vi "pmu_Write ROCOF Detector Settings.vi"(8 "error in (no error)":errorcluster, 10 "ROCOF detector settings":T1={"ROCOF window width"=2}, 11 "system info in":refnum<class "PMU System Info.lvclass">) -> (0 "error out":errorcluster, 3 "system info out":refnum<class "PMU System Info.lvclass">)   [LabVIEW 2013, in "NI_EP_PMU.lvlib" / "PMU System Info.lvclass"]
uses:
  <vilib>/addons/Electrical Power/PMU/Common/Classes/PMU System Info/PMU System Info.lvclass
  <vilib>/addons/Electrical Power/PMU/Common/Controls/pmu_ROCOF Detector Settings.ctl
  <vilib>/addons/Electrical Power/PMU/Common/Classes/PMU System Info/PMU System Info.lvclass/PMU System Info.ctl
  <vilib>/addons/Electrical Power/PMU/NI_EP_PMU.lvlib
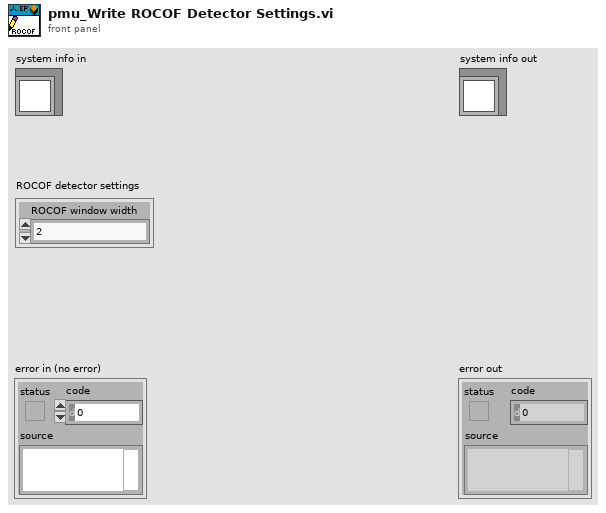
[diagram p1: front panel]
types:
  T1 = typedef "NI_EP_PMU.lvlib/pmu_ROCOF Detector Settings.ctl" = cluster{"ROCOF window width":i32}
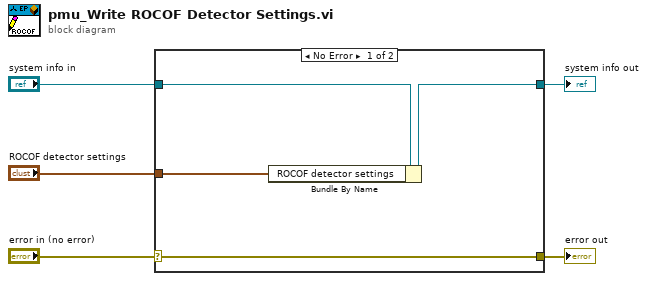
[diagram p0: block diagram]
diagram:
  n1 = case shown="No Error" "error in (no error)" {
    selector: "error in (no error)" -> [w9 w10]
    tunnel: [w9 w10] -> w4
    tunnel: [w7 w11] -> w2
    tunnel: "system info in" -> [w8 w11]
    tunnel: "ROCOF detector settings" -> [w6 _]
    frame No Error {
      n2 = Bundle By Name(cluster=w8, "ROCOF detector settings"=w6) -> (w7:refnum<class "PMU System Info.lvclass">)
    }
    frame Error {
    }
  }
  "error out" <- w4
  "system info out" <- w2
